vi "General PID Simulator_DEMO.vi"() -> ()   [LabVIEW 2010]
panel:
  in  "STOP":bool
  in  "process parameters":T1={"static gain"=2.5, "lag (min)"=0.3, "dead cycles"=1, "load %"=40.0, "deadband"=2.0, "noise level %"=0.25, "initial PV"=0.0} {"initial PV" format="%.2f"; "noise level %" format="%.2f"; "lag (min)" format="%.2f"; "dead cycles" format="%.2f"; "deadband" format="%.1f"; "load %" format="%.2f"; "static gain" format="%.2f"}
  out "PV Setpoint Output":T2(graph)={"initial PV"=18.934717983735947, "SP(%)"=34.59119496855346, "output"=100.0}
  in  "Sampling Time dt (s)":dbl=0.05 min=0.001 step=0.01 format="%#.3p"
  in  "PID gains":T3={"proportional gain (Kc)"=20.0, "integral time (Ti, min)"=0.008, "derivative time (Td, min)"=0.001} {"derivative time (Td, min)" format="%.3f"; "integral time (Ti, min)" format="%.3f"; "proportional gain (Kc)" format="%.3f"}
  out "PV:":dbl(slide)=60.754431603254424 scale=0.0..100.0
  in  "SP:":dbl(slide)=60.7843137254902 min=0.0 max=0.0 scale=0.0..100.0
  out "MV:":dbl(slide)=18.78965245852964 scale=-100.0..100.0
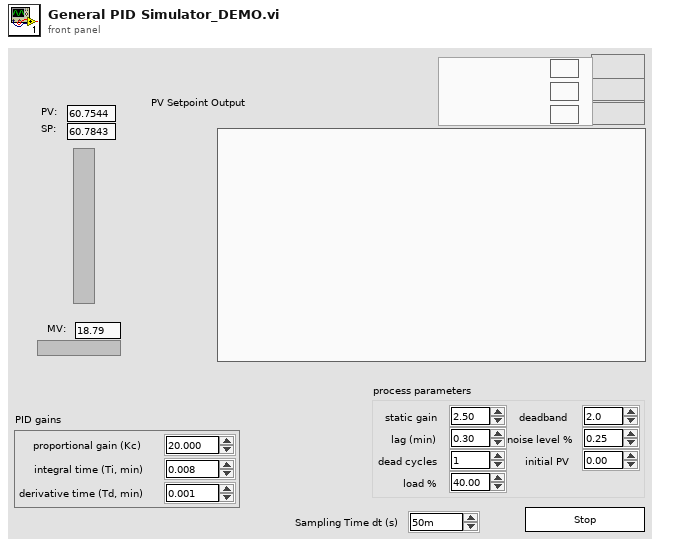
[diagram p1: front panel]
types:
  T1 = cluster{"static gain":dbl, "lag (min)":dbl, "dead cycles":i32, "load %":dbl, "deadband":dbl, "noise level %":dbl, "initial PV":dbl}
  T2 = cluster{"initial PV":dbl, "SP(%)":dbl, "output":dbl}
  T3 = cluster{"proportional gain (Kc)":dbl, "integral time (Ti, min)":dbl, "derivative time (Td, min)":dbl}
  T4 = cluster{"initial PV":dbl, "SP:":dbl, "output":dbl}
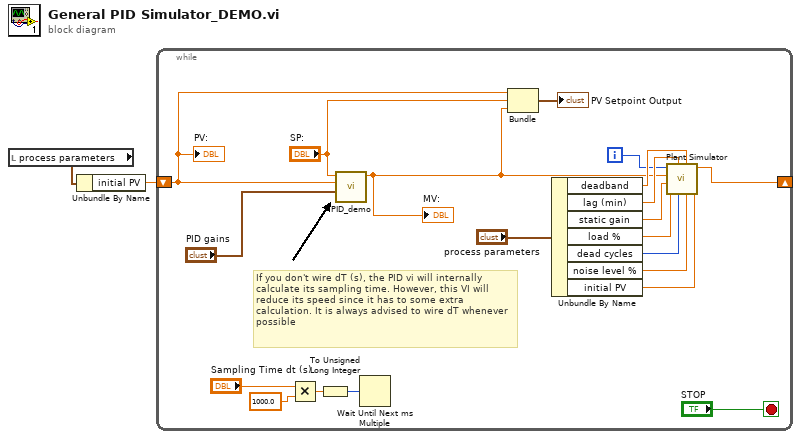
[diagram p0: block diagram]
diagram:
  n1 = local read "process parameters"() -> (w1:T1)
  n2 = Unbundle By Name(w1) -> ("initial PV"=w2:dbl)
  n3 = while {
    shift-left: w2 -> [w7]
    shift-right: [w12] -> _
    i -> [w10]
    stop <- "STOP" stop-if-true
    # "If you don't wire dT (s), the PID vi will internally calculate its sampling time. However, this VI will reduce its speed since it has to some extra calculation. It is always advised to wire dT whenever possible"
    n4 = Multiply(x="Sampling Time dt (s)", y=1000.0) -> (x*y=w21:dbl)
    n5 = To Unsigned Long Integer(number=w21) -> (unsigned 32bit integer=w15:u32)
    n6 = call "PID_demo.vi"("PID gains"="PID gains", "process variable"=w7, "setpoint"="SP:") -> ("output"=w5:dbl)  [unwired: 7 in, 1 out]
    "MV:" <- w5
    n7 = Wait Until Next ms Multiple(millisecond multiple=w15) -> ()  [unwired: 1 out]
    n8 = Bundle("initial PV"=w7, "SP:"="SP:", "output"=w5) -> (→"PV Setpoint Output":T4)  [unwired: 1 in]
    n9 = Unbundle By Name("process parameters") -> ("deadband"=w19:dbl, "lag (min)"=w13:dbl, "static gain"=w18:dbl, "load %"=w17:dbl, "dead cycles"=w3:i32, "noise level %"=w14:dbl, "initial PV"=w11:dbl)
    n10 = call "Plant Simulator.vi"("Initial PV"=w11, "Controller Noise (%)"=w14, "Valve Deadband"=w19, "Process Deadtime"=w3, "Lag (min)"=w13, "Process Load"=w17, "Process Gain"=w18, "Manipulated Variable (Output, %)"=w5, "iteration"=w10) -> ("Process Variable (%)"=w12:dbl)  [unwired: 2 in]
    "PV:" <- w7
  }
